vi "Serial Port Monitor.vi"() -> ()   [LabVIEW 2023]
doc: "This example allows the user to monitor the serial lines. The 2 output lines that can be written to are DTR and RTS. The 4 input lines are DCD, RI, DSR and CTS. This example can be run alongside another example or VI talking to the same port. This example is intended for troubleshooting purposes.\n\nTo test the lines, you can also run this example alone with the following connections. Short pin 4 to pin 6 (DTR/DSR) or pin 7 to pin 8 (RTS/CTS) for RS-232. For RS-485, short pin 2 to pin 3 (CTS+/RTS+) and short pin 6 to pin 7 (CTS-/RTS-). If you specify TRUE values for both \"DTR Write\" and \"RTS Write\", you can see the corresponding handshaking lines turn on and off when you change the DTR and RTS values.\n\nWhen running a handshaking application with an instrument, you may want to monitor the state of the lines to verify that the handshaking is operating as expected. Alternatively, if your application is not communicating as expected, this example allows you to view exactly what is happening with the lines."
panel:
  in  "Stop":bool
  out "CTS":bool=TRUE
  out "DSR":bool
  out "RI":bool
  out "DCD":bool
  out "RTS":bool
  in  "RTS Write":bool
  out "DTR":bool
  in  "DTR Write":bool
  in  "Serial Port":refnum<visa-resource-name>="COM1"
  # "Overview: Demonstrates the use of the VISA functions to monitor the Serial port.\nRequirements: NI-VISA Driver\nInstructions:\n1. Ensure the Serial Port value is valid.\n2. Run the VI.\n3. Observe the serial port status displayed by the LEDs.\n4. Set the DTR and RTS values with their respective push buttons, and observe their values reflected in the LEDs.\n5. Click Stop to stop the VI."
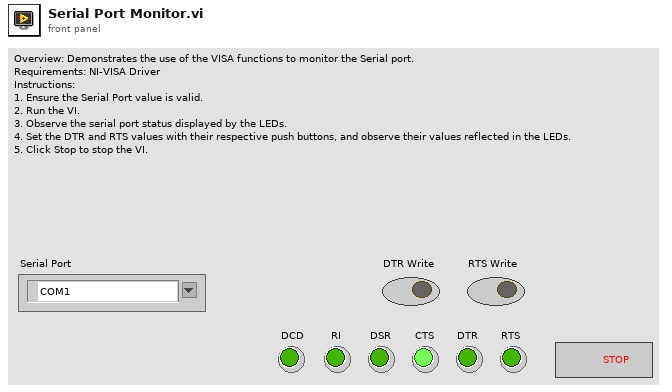
[diagram p1: front panel]
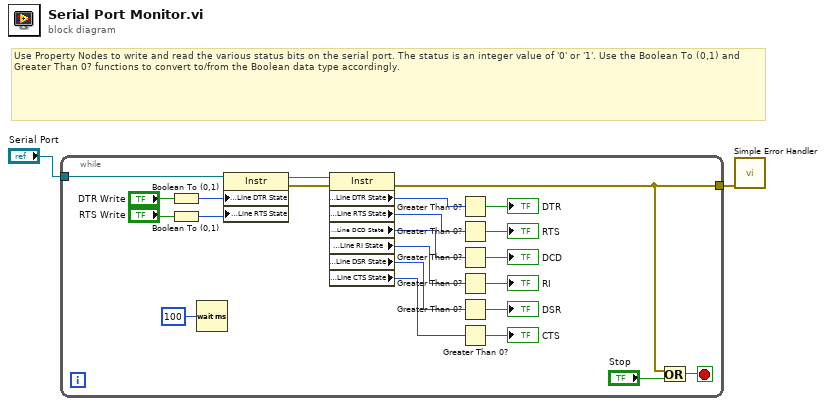
[diagram p0: block diagram]
diagram:
  # "Use Property Nodes to write and read the various status bits on the serial port. The status is an integer value of '0' or '1'. Use the Boolean To (0,1) and Greater Than 0? functions to convert to/from the Boolean data type accordingly."
  n1 = while {
    tunnel: "Serial Port" -> [w24]
    tunnel: [w7] -> w1
    stop <- w25 stop-if-true
    n2 = Boolean To (0,1)(Boolean="DTR Write") -> (0, 1=w3:i16)
    n3 = Boolean To (0,1)(Boolean="RTS Write") -> (0, 1=w5:i16)
    n4 = Wait (ms)(milliseconds to wait=u32 100 ("millisecond multiple")) -> ()  [unwired: 1 out]
    n5 = property class="Instr"(reference=w24, "Serial Settings:Modem Line Settings:Line DTR State"=w3, "Serial Settings:Modem Line Settings:Line RTS State"=w5) -> (reference out=w23:refnum<visa-resource-name>, error out=w22:errorcluster)  [unwired: 1 in]
    n6 = property class="Instr"(reference=w23, error in=w22) -> (error out=w7:errorcluster, "Serial Settings:Modem Line Settings:Line DTR State"=w18:i16, "Serial Settings:Modem Line Settings:Line RTS State"=w15:i16, "Serial Settings:Modem Line Settings:Line DCD State"=w16:i16, "Serial Settings:Modem Line Settings:Line RI State"=w21:i16, "Serial Settings:Modem Line Settings:Line DSR State"=w20:i16, "Serial Settings:Modem Line Settings:Line CTS State"=w19:i16)  [unwired: 1 out]
    n7 = Greater Than 0?(x=w18) -> (x > 0?=→"DTR":bool)
    n8 = Greater Than 0?(x=w15) -> (x > 0?=→"RTS":bool)
    n9 = Greater Than 0?(x=w16) -> (x > 0?=→"DCD":bool)
    n10 = Greater Than 0?(x=w21) -> (x > 0?=→"RI":bool)
    n11 = Greater Than 0?(x=w20) -> (x > 0?=→"DSR":bool)
    n12 = Greater Than 0?(x=w19) -> (x > 0?=→"CTS":bool)
    n13 = Or(x=w7, y="Stop") -> (x .or. y?=w25:bool)
  }
  n14 = call <vilib>:"Simple Error Handler.vi"("error in (no error)"=w1) -> ()  [unwired: 1 in, 8 out]
